vi "Main.vi"(8 "Error In":errorcluster, 11 "new reference":refnum<k24>) -> ()   [LabVIEW 2019]
uses:
  Microsoft.Office.Interop.Excel
  <vilib>/Analysis/NI_AALBase.lvlib
panel:
  out "Waveform Chart":dbl[](graph)
  out "Boolean":bool
  in  "Stop":bool
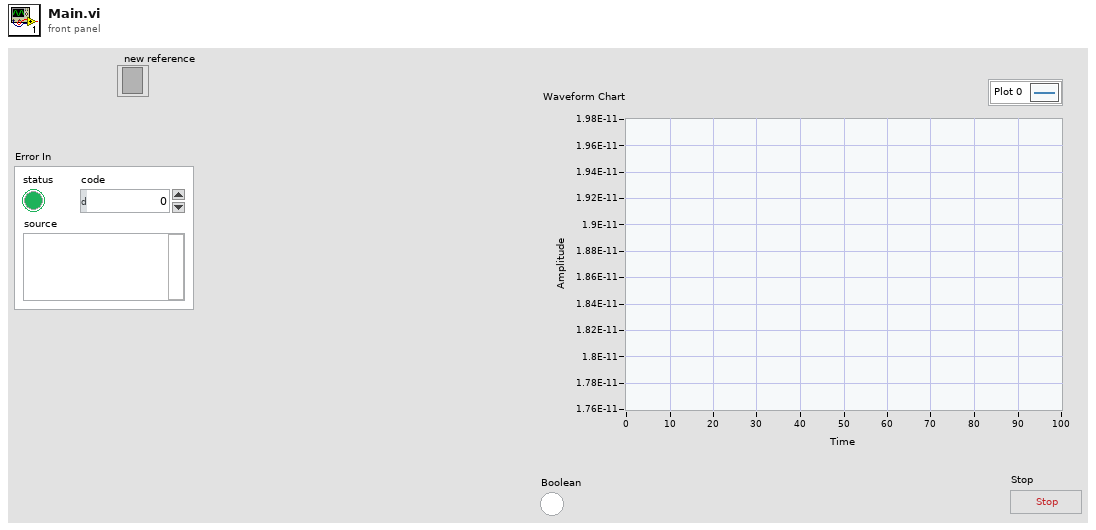
[diagram p1: front panel]
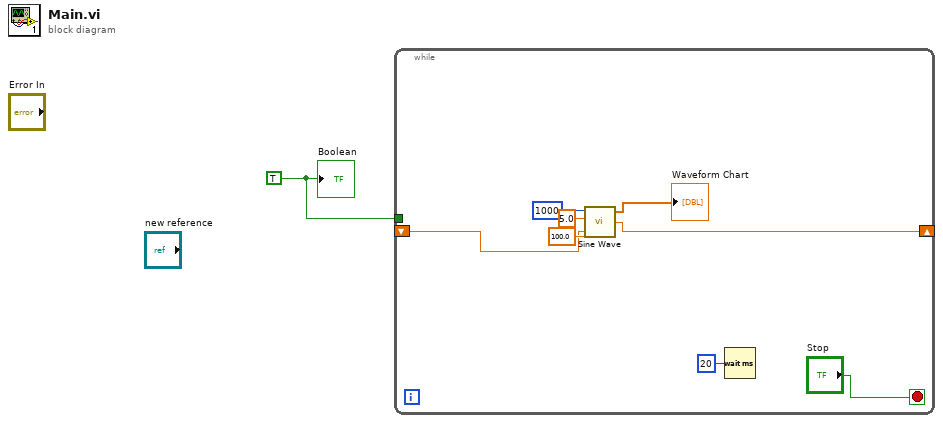
[diagram p0: block diagram]
diagram:
  w1 = TRUE
  n1 = while {
    tunnel: w1 -> [_]
    shift-right: [w3] -> _
    shift-left: _ -> [w2]
    stop <- "Stop" stop-if-true
    n2 = call <vilib>:"Sine Wave.vi"("samples"=1000, "amplitude"=5.0, "frequency"=100.0, "phase in"=w2) -> ("sine wave"=→"Waveform Chart":dbl[], "phase out"=w3:dbl)  [unwired: 1 in, 1 out]
    n3 = Wait (ms)(milliseconds to wait=u32 20) -> ()  [unwired: 1 out]
  }
  "Boolean" <- w1
